vi "Download Worker.vi"(8 "Error In":errorcluster, 11 "Download":T1) -> (0 "Error Out":errorcluster, 3 "Download":T1)   [LabVIEW 2014, in "LMH-Toolbox.lvlib" / "LMH-Web.lvlib"]
uses:
  <vilib>/MakerHub/Toolbox/Private/Web/LMH-Web.lvlib
  <vilib>/MakerHub/Toolbox/Private/Web/Type Defs/Download Task.ctl
  <vilib>/httpClient/LabVIEWHTTPClient.lvlib
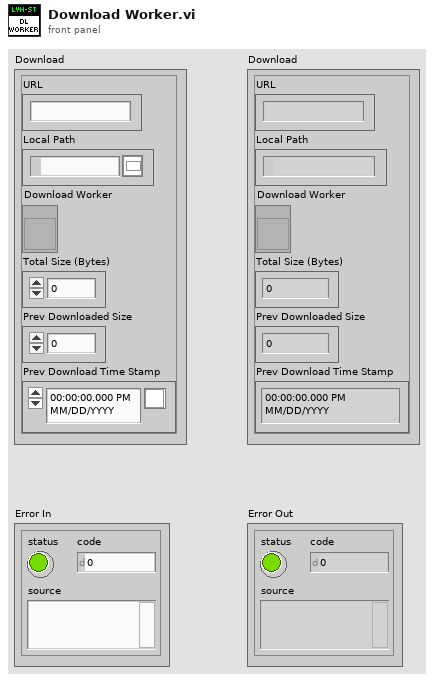
[diagram p1: front panel]
types:
  T1 = typedef "LMH-Toolbox.lvlib/LMH-Web.lvlib/Download Task.ctl" = cluster{"URL":string, "Local Path":path, "Download Worker":refnum<vi>, "Total Size (Bytes)":u64, "Prev Downloaded Size":u64, "Prev Download Time Stamp":timestamp}
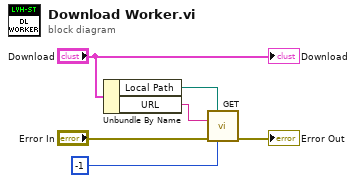
[diagram p0: block diagram]
diagram:
  n1 = Unbundle By Name("Download") -> ("Local Path"=w5:path, "URL"=w4:string)
  n2 = call <vilib>:"GET.vi"("output file"=w5, "url"=w4, "error in (no error)"="Error In", "timeout (10000)"=-1) -> ("error out"=→"Error Out":errorcluster)  [unwired: 8 in, 3 out]
  "Download" <- "Download"
